vi "After Run TS.vi"(8 "error in":errorcluster, 11 "Heat Flow Test Stand in":refnum<class "Heat Flow Test Stand.lvclass">) -> (0 "error out":errorcluster, 3 "Heat Flow Test Stand out":refnum<class "Heat Flow Test Stand.lvclass">)   [LabVIEW 2019, in "Test Stands.lvlib" / "Heat Flow Test Stand.lvclass"]
uses:
  Heat Flow Test Stand.lvclass
  DAC/Heat Flow/HeatFlow AIV/DAC HeatFlow AIV.lvclass
  Generic Test Stand/Generic Test Stand.lvclass
  DAC/DAC.lvclass
  C:/Users/wg/Documents/LV_Projects/test-stand/App/Generic Test Stand/Generic Test Stand.lvclass
  C:/Users/wg/Documents/LV_Projects/test-stand/App/DAC/DAC.lvclass
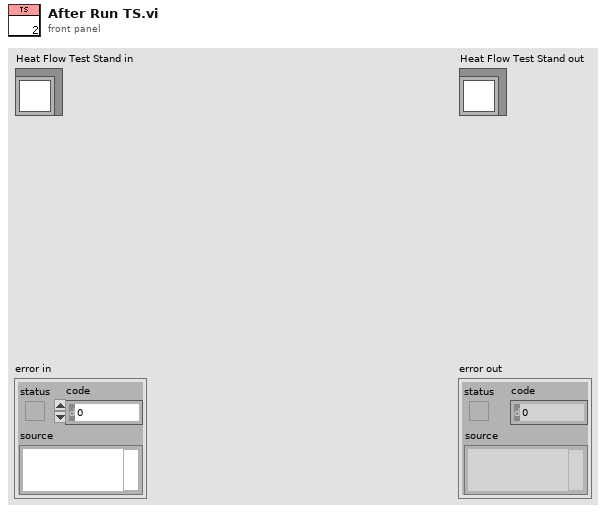
[diagram p1: front panel]
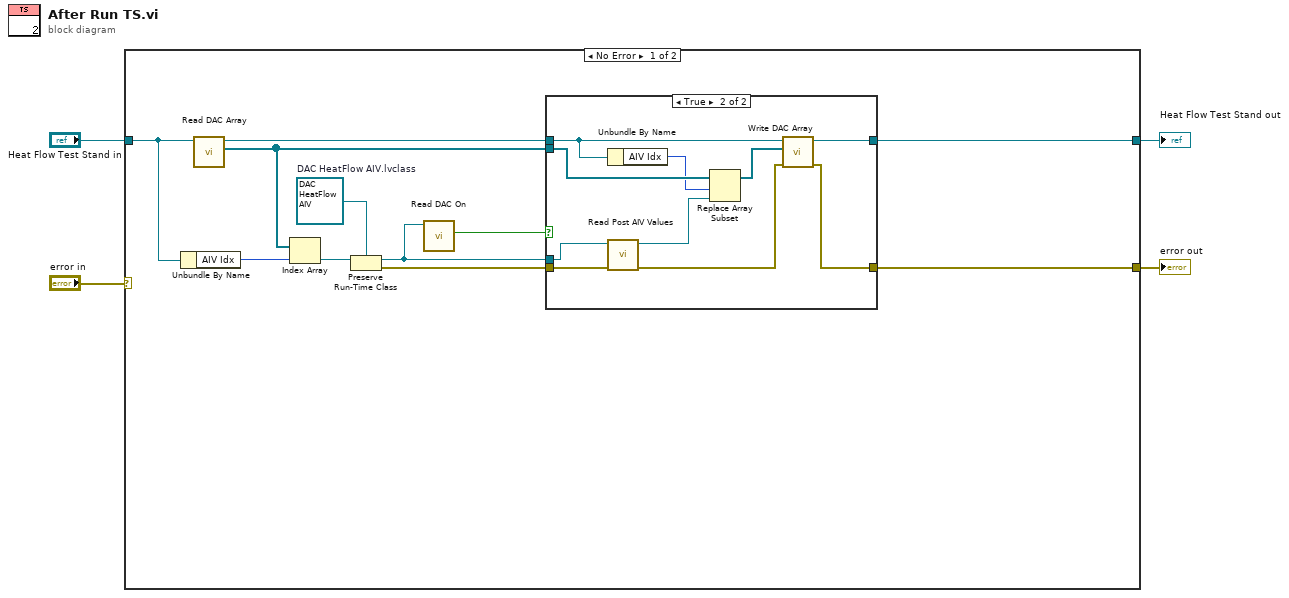
[diagram p0: block diagram]
diagram:
  n1 = case shown="No Error" "error in" {
    selector: "error in" -> [_ w29]
    tunnel: [w5 w29] -> w1
    tunnel: [w6 w28] -> w2
    tunnel: "Heat Flow Test Stand in" -> [w9 w28]
    frame No Error {
      w8 = refnum<class "DAC HeatFlow AIV.lvclass"> refnum  # DAC HeatFlow AIV.lvclass
      n2 = Unbundle By Name(w9) -> ("AIV Idx"=w13:i32)
      n3 = call "Read DAC Array.vi"("Generic Test Stand in"=w9) -> ("DAC Array"=w10:refnum<class "DAC.lvclass">[], "Generic Test Stand out"=w14:refnum<class "Heat Flow Test Stand.lvclass">)  [unwired: 8 in, 1 out]
      n4 = Index Array(array=w10, index=w13) -> (element=w12:refnum<class "DAC.lvclass">)
      n5 = Preserve Run-Time Class(object in=w12, 2:w8) -> (object out=w7:refnum<class "DAC HeatFlow AIV.lvclass">, error out=w11:errorcluster)  [unwired: 1 in]
      n6 = call "Read DAC On.vi"("DAC in"=w7) -> ("DAC On"=w15:bool)  [unwired: 8 in, 2 out]
      n7 = case shown="True" w15 {
        tunnel: w14 -> [w17 w25]
        tunnel: [w17 w27] -> w6
        tunnel: w7 -> [_ w20]
        tunnel: w11 -> [w16 w21]
        tunnel: w10 -> [_ w26]
        tunnel: [w16 w22] -> w5
        frame False {
        }
        frame True {
          n8 = Unbundle By Name(w25) -> ("AIV Idx"=w24:i32)
          n9 = call "Read Post AIV Values.vi"("error in"=w21, "DAC HeatFlow AIV in"=w20) -> ("error out"=w18:errorcluster, "DAC HeatFlow AIV out"=w19:refnum<class "DAC HeatFlow AIV.lvclass">)  [unwired: 8 in]
          n10 = Replace Array Subset(array=w26, new element=w19, index=w24) -> (w23:refnum<class "DAC.lvclass">[])
          n11 = call "Write DAC Array.vi"("error in (no error)"=w18, "DAC Array"=w23, "Generic Test Stand in"=w25) -> ("error out"=w22:errorcluster, "Generic Test Stand out"=w27:refnum<class "Heat Flow Test Stand.lvclass">)  [unwired: 7 in]
        }
      }
    }
    frame Error {
    }
  }
  "error out" <- w1
  "Heat Flow Test Stand out" <- w2
